vi "testExample 7.vi"(8 "error in (no error)":errorcluster, 11 "TestCase in":refnum<class "Test simulado.lvclass">) -> (0 "error out":errorcluster, 3 "TestCase out":refnum<class "Test simulado.lvclass">)   [LabVIEW 2020, in "Test simulado.lvclass"]
doc: "Este VI TEST es para las pruebas del Serial Device simulado.\nLas pruebas a las que está sometido son:\nADC Read\nGet Port\nSet Port\nGet Pin\nSet Pin"
uses:
  Test simulado.lvclass
  Implementation/Simulado/Simulado.lvclass
  <vilib>/addons/_JKI Toolkits/VI Tester/TestCase.llb/TestCase.lvclass
  UI Actor/UI Actor.lvclass
  C:/Program Files (x86)/National Instruments/LabVIEW 2020/vi.lib/addons/_JKI Toolkits/VI Tester/TestCase.llb/TestCase.lvclass
panel:
  out "ADC":dbl
  in  "Read ADC":bool
  out "Valor pin":string
  out "Pin":string
  out "Puerto":string
  in  "PIN":i32
  in  "Valor pin":string(combo)
  in  "Set Pin":bool
  in  "Get Pin":bool
  in  "Byte 0":string(combo)
  in  "Byte 1":string(combo)
  in  "CH":i32
  in  "Seleccion de prueba":string(combo)
  in  "Set Port":bool
  out "Leds":bool[](array[boolean])
  in  "Buttons":bool[](array[boolean])
  in  "Get Port":bool
  in  "Conexión simulada":bool
  out "Simulado out":refnum<class "Simulado.lvclass">
  in  "Simulado in":refnum<class "Simulado.lvclass">
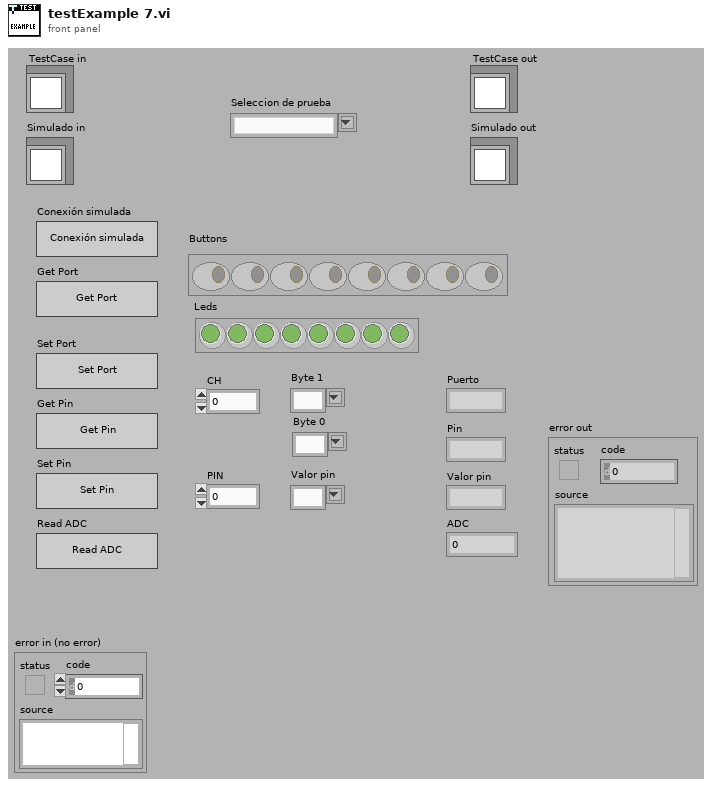
[diagram p1: front panel]
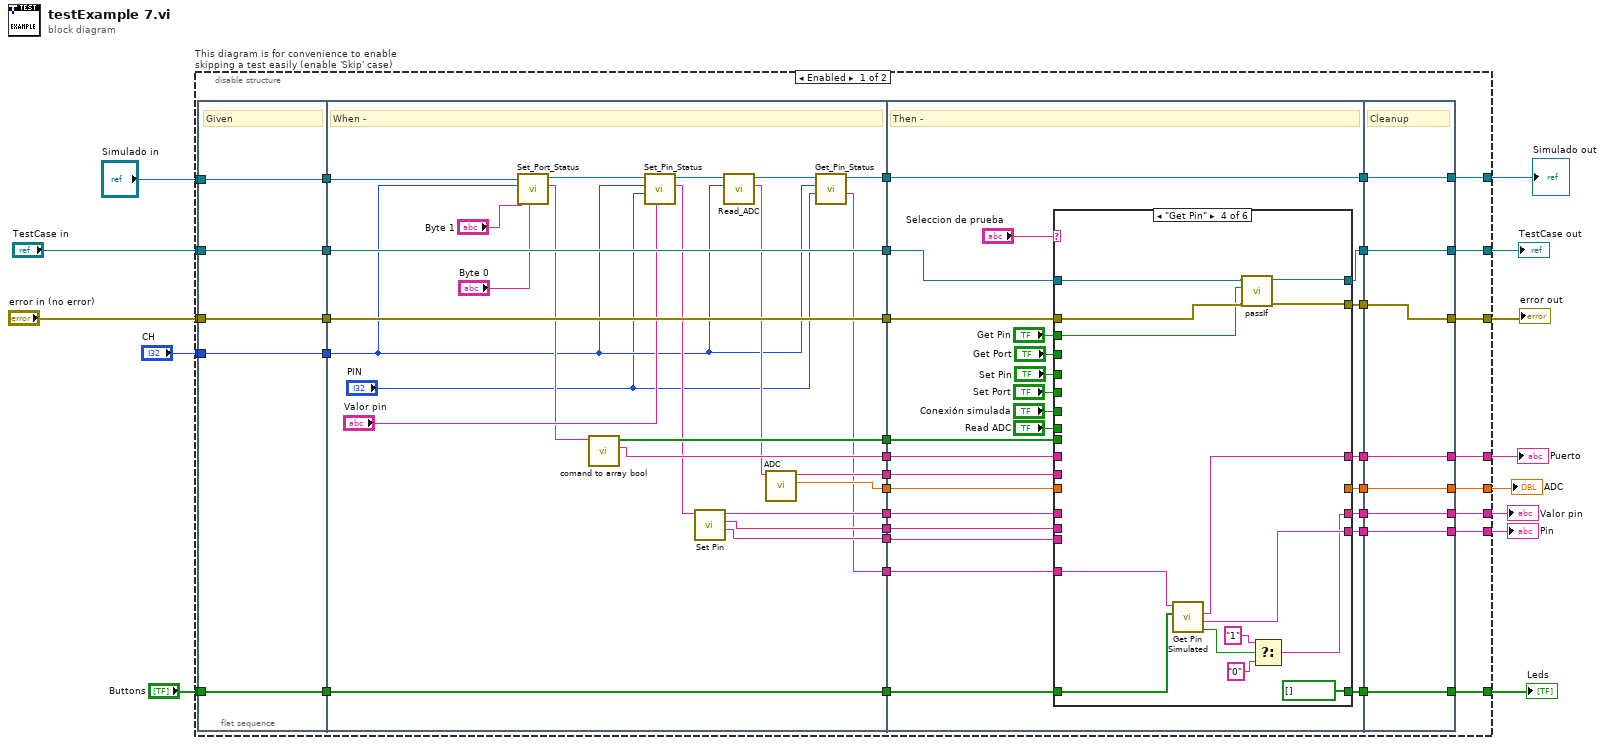
[diagram p0: block diagram]
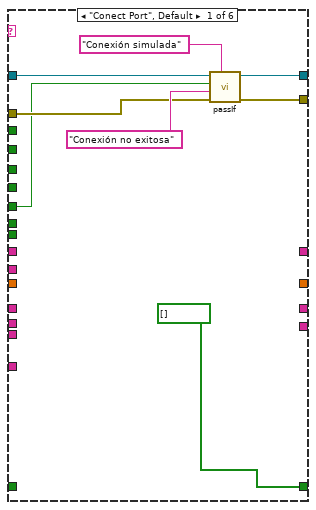
[diagram p2: hidden frame]
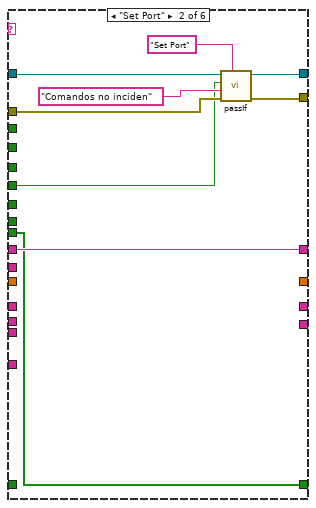
[diagram p3: hidden frame]
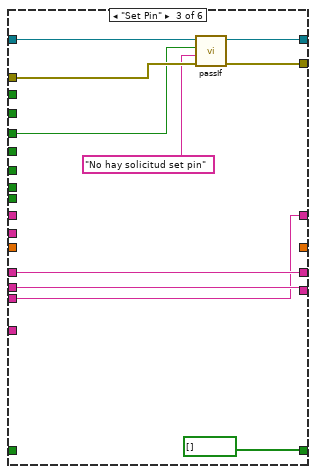
[diagram p4: hidden frame]
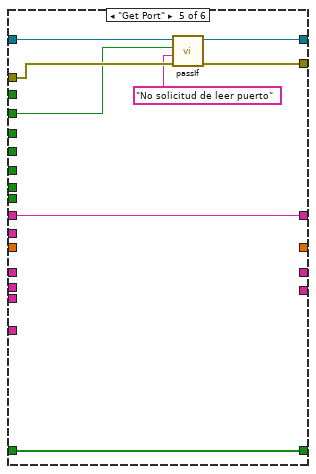
[diagram p5: hidden frame]
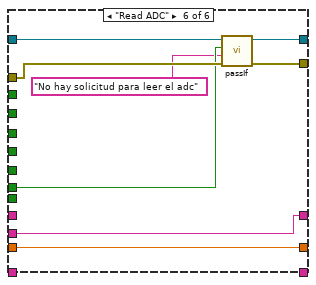
[diagram p6: hidden frame]
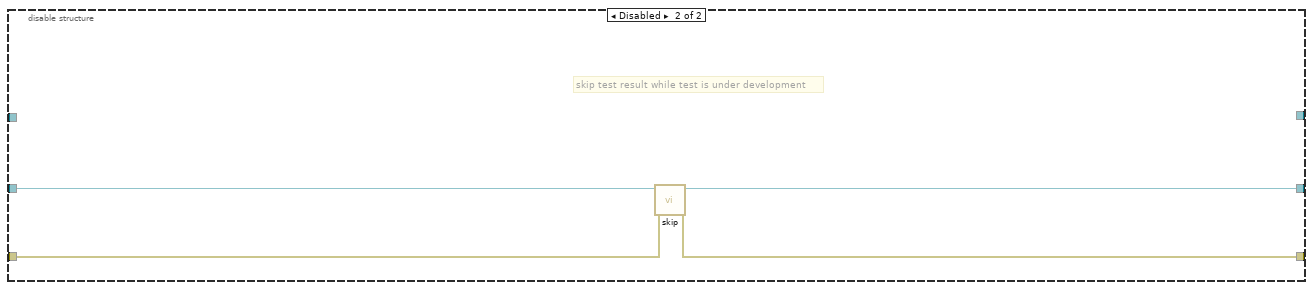
[diagram p7: hidden frame]
diagram:
  n1 = disable-structure "This diagram is for convenience to enable skipping a test easily (enable 'Skip' case)" shown="Enabled" {
    disable-tunnel: "TestCase in" -> [w45 w175]
    disable-tunnel: [w43 w173] -> w10
    disable-tunnel: [w42 w174] -> w12
    disable-tunnel: "error in (no error)" -> [w44 w172]
    disable-tunnel: "Simulado in" -> [w39 _]
    disable-tunnel: [w37 _] -> w8
    disable-tunnel: "Buttons" -> [w35 _]
    disable-tunnel: [w34 _] -> w6
    disable-tunnel: "CH" -> [w30 _]
    disable-tunnel: [w27 _] -> w4
    disable-tunnel: [w25 _] -> w3
    disable-tunnel: [w22 _] -> w2
    disable-tunnel: [w15 _] -> w1
    frame Enabled {
      n2 = flat-sequence {
        tunnel: w44 -> [w55]
        tunnel: w45 -> [w56]
        tunnel: [w56] -> w51
        tunnel: [w55] -> w50
        tunnel: [w54] -> w40
        tunnel: w39 -> [w54]
        tunnel: [w53] -> w36
        tunnel: w35 -> [w53]
        tunnel: [w52] -> w31
        tunnel: w30 -> [w52]
        tunnel: [w80] -> w49
        tunnel: [w79] -> w48
        tunnel: w51 -> [w80]
        tunnel: w50 -> [w79]
        tunnel: [w60] -> w41
        tunnel: w40 -> [w77]
        tunnel: w36 -> [w78]
        tunnel: [w78] -> w32
        tunnel: w31 -> [w59]
        tunnel: [w74] -> w29
        tunnel: [w70] -> w28
        tunnel: [w68] -> w23
        tunnel: [w67] -> w20
        tunnel: [w66] -> w19
        tunnel: [w63] -> w18
        tunnel: [w62] -> w17
        tunnel: [w57] -> w14
        tunnel: [w104] -> w47
        tunnel: [w105] -> w46
        tunnel: w49 -> [w102]
        tunnel: w48 -> [w103]
        tunnel: w41 -> [w106]
        tunnel: [w106] -> w38
        tunnel: [w100] -> w33
        tunnel: w32 -> [w99]
        tunnel: w29 -> [w98]
        tunnel: w28 -> [w94]
        tunnel: [w93] -> w26
        tunnel: [w90] -> w24
        tunnel: w23 -> [w89]
        tunnel: [w88] -> w21
        tunnel: w20 -> [w87]
        tunnel: w19 -> [w86]
        tunnel: w18 -> [w84]
        tunnel: w17 -> [w83]
        tunnel: [w82] -> w16
        tunnel: w14 -> [w81]
        tunnel: [w170] -> w42
        tunnel: [w171] -> w43
        tunnel: w47 -> [w171]
        tunnel: w46 -> [w170]
        tunnel: [w169] -> w37
        tunnel: w38 -> [w169]
        tunnel: [w168] -> w34
        tunnel: w33 -> [w168]
        tunnel: [w167] -> w27
        tunnel: w26 -> [w167]
        tunnel: [w166] -> w25
        tunnel: w24 -> [w166]
        tunnel: [w165] -> w22
        tunnel: w21 -> [w165]
        tunnel: w16 -> [w164]
        tunnel: [w164] -> w15
        frame #0 {
          # "Given"
        }
        frame #1 {
          # "When -"
          n3 = call-dynamic "Set_Port_Status.vi"("Byte 0"="Byte 0", "Byte 1"="Byte 1", "CH"=w59, "Simulado in"=w77) -> ("Command to Send"=w71:string, "Simulado out"=w73:refnum<class "Simulado.lvclass">)  [unwired: 4 in, 2 out]
          n4 = call "comand to array bool.vi"("Command to Send"=w71) -> ("Puerto"=w70:string, "output array"=w74:bool[])  [unwired: 9 in]
          n5 = call-dynamic "Set_Pin_Status.vi"("Valor pin"="Valor pin", "PIN"="PIN", "CH"=w59, "Simulado in"=w73) -> ("Command to Send"=w69:string, "Simulado out"=w65:refnum<class "Simulado.lvclass">)  [unwired: 4 in, 2 out]
          n6 = call "Set Pin.vi"("Command to Send"=w69) -> ("Puerto"=w66:string, "Pin"=w67:string, "Valor pin"=w68:string)  [unwired: 8 in]
          n7 = call-dynamic "Read_ADC.vi"("CH"=w59, "Simulado in"=w65) -> ("Command to Send"=w64:string, "Simulado out"=w61:refnum<class "Simulado.lvclass">)  [unwired: 6 in, 2 out]
          n8 = call "ADC.vi"("Command to Send"=w64) -> ("ADC"=w62:dbl, "Puerto"=w63:string)  [unwired: 9 in]
          n9 = call-dynamic "Get_Pin_Status.vi"("PIN"="PIN", "CH"=w59, "Simulado in"=w61) -> ("Expected Response"=w57:string, "Simulado out"=w60:refnum<class "Simulado.lvclass">)  [unwired: 5 in, 2 out]
        }
        frame #2 {
          # "Then -"
          n10 = case shown="\"Get Pin\"" "Seleccion de prueba" {
            tunnel: w102 -> [w111 w121 w133 w147 w155 w163]
            tunnel: [w110 w119 w132 w145 w154 w160] -> w104
            tunnel: w103 -> [w112 w120 w131 w146 w152 w162]
            tunnel: [w109 w118 w130 w144 w153 w161] -> w105
            tunnel: [bool[] [] ("Leds") w115 bool[] [] ("Buttons") bool[] [] ("Buttons") w150 _] -> w100
            tunnel: w99 -> [_ _ _ w141 w150 _]
            tunnel: w98 -> [_ w115 _ _ _ _]
            tunnel: "Conexión simulada" -> [w107 _ _ _ _ _]
            tunnel: "Set Port" -> [_ w117 _ _ _ _]
            tunnel: "Set Pin" -> [_ _ w129 _ _ _]
            tunnel: w94 -> [_ w116 _ _ w149 _]
            tunnel: [_ w116 w124 w139 w149 w157] -> w93
            tunnel: "Get Pin" -> [_ _ _ w143 _ _]
            tunnel: "Get Port" -> [_ _ _ _ w148 _]
            tunnel: [_ _ w126 w134 _ _] -> w90
            tunnel: w89 -> [_ _ w126 _ _ _]
            tunnel: [_ _ w125 w138 _ _] -> w88
            tunnel: w87 -> [_ _ w125 _ _ _]
            tunnel: w86 -> [_ _ w124 _ _ _]
            tunnel: "Read ADC" -> [_ _ _ _ _ w159]
            tunnel: w84 -> [_ _ _ _ _ w157]
            tunnel: w83 -> [_ _ _ _ _ w156]
            tunnel: [_ _ _ _ _ w156] -> w82
            tunnel: w81 -> [_ _ _ w140 _ _]
            frame "Conect Port", Default {
              n11 = call-dynamic "passIf.vi"("custom report message (\"\")"="Conexión simulada" ("custom report message (\"\")"), "error in (no error)"=w112, "message (\"\")"="Conexión no exitosa" ("message (\"\")"), "pass"=w107, "TestCase in"=w111) -> ("error out"=w109:errorcluster, "TestCase out"=w110:refnum<class "Test simulado.lvclass">)  [unwired: 5 in]
            }
            frame "Set Port" {
              n12 = call-dynamic "passIf.vi"("custom report message (\"\")"="Set Port" ("custom report message (\"\")"), "error in (no error)"=w120, "message (\"\")"="Comandos no inciden" ("message (\"\")"), "pass"=w117, "TestCase in"=w121) -> ("error out"=w118:errorcluster, "TestCase out"=w119:refnum<class "Test simulado.lvclass">)  [unwired: 5 in]
            }
            frame "Set Pin" {
              n13 = call-dynamic "passIf.vi"("error in (no error)"=w131, "message (\"\")"="No hay solicitud set pin" ("message (\"\")"), "pass"=w129, "TestCase in"=w133) -> ("error out"=w130:errorcluster, "TestCase out"=w132:refnum<class "Test simulado.lvclass">)  [unwired: 6 in]
            }
            frame "Get Pin" {
              n14 = call "Get Pin Simulated.vi"("Buttons"=w141, "Exprected Response"=w140) -> ("Valor pin"=w137:bool, "PIN"=w138:string, "Port"=w139:string)  [unwired: 6 in, 1 out]
              n15 = call-dynamic "passIf.vi"("error in (no error)"=w146, "pass"=w143, "TestCase in"=w147) -> ("error out"=w144:errorcluster, "TestCase out"=w145:refnum<class "Test simulado.lvclass">)  [unwired: 7 in]
              n16 = Select(t="1", s=w137, f="0") -> (s? t:f=w134:string)
            }
            frame "Get Port" {
              n17 = call-dynamic "passIf.vi"("error in (no error)"=w152, "message (\"\")"="No solicitud de leer puerto" ("message (\"\")"), "pass"=w148, "TestCase in"=w155) -> ("error out"=w153:errorcluster, "TestCase out"=w154:refnum<class "Test simulado.lvclass">)  [unwired: 6 in]
            }
            frame "Read ADC" {
              n18 = call-dynamic "passIf.vi"("error in (no error)"=w162, "message (\"\")"="No hay solicitud para leer el adc" ("message (\"\")"), "pass"=w159, "TestCase in"=w163) -> ("error out"=w161:errorcluster, "TestCase out"=w160:refnum<class "Test simulado.lvclass">)  [unwired: 6 in]
            }
          }
        }
        frame #3 {
          # "Cleanup"
        }
      }
    }
    frame Disabled {
      # "skip test result while test is under development"
      n19 = call <vilib>:"skip.vi"("error in (no error)"=w172, "TestCase in"=w175) -> ("error out"=w174:errorcluster, "TestCase out"=w173:refnum<class "Test simulado.lvclass">)  [unwired: 8 in]
    }
  }
  "error out" <- w12
  "TestCase out" <- w10
  "Simulado out" <- w8
  "Leds" <- w6
  "Puerto" <- w4
  "Pin" <- w2
  "Valor pin" <- w3
  "ADC" <- w1
